vi "SetStringLength.vi"(2 "Input String":string, 3 "String Length":i32) -> (1 "Output String":string)   [LabVIEW 2022 SP3]
panel:
  out "length":i32
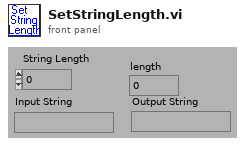
[diagram p1: front panel]
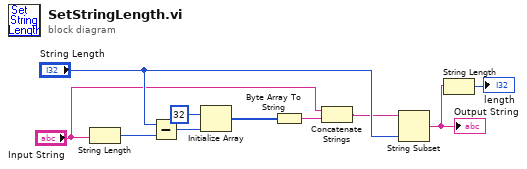
[diagram p0: block diagram]
diagram:
  n1 = String Length(string="Input String") -> (length=w7:i32)
  n2 = Subtract(x="String Length", y=w7) -> (x-y=w6:i32)
  n3 = Initialize Array(u8 32, w6) -> (w4:u8[])
  n4 = Byte Array To String(unsigned byte array=w4) -> (string=w2:string)
  n5 = Concatenate Strings("Input String", w2) -> (w1:string)
  n6 = String Subset(string=w1, length (rest)="String Length") -> (substring=w10:string)  [unwired: 1 out]
  "Output String" <- w10
  n7 = String Length(string=w10) -> (length=→"length":i32)
